vi "Write Close Panel on Exit_.vi"(8 "error in (no error)":errorcluster, 10 "Close Panel on Exit?":bool, 11 "UI ActorTop in":refnum<class "UIActorTop.lvclass">) -> (0 "error out":errorcluster, 3 "UI ActorTop out":refnum<class "UIActorTop.lvclass">)   [LabVIEW 2021, in "AbstractActorTemplate.lvlib" / "UIActorTop.lvclass"]
uses:
  <userlib>/John_Lib/AbstractActorTemplate/AbstractActorTemplate/UIActorTop.lvclass
  <userlib>/John_Lib/AbstractActorTemplate/AbstractActorTemplate/UIActorTop.lvclass/UIActorTop.ctl
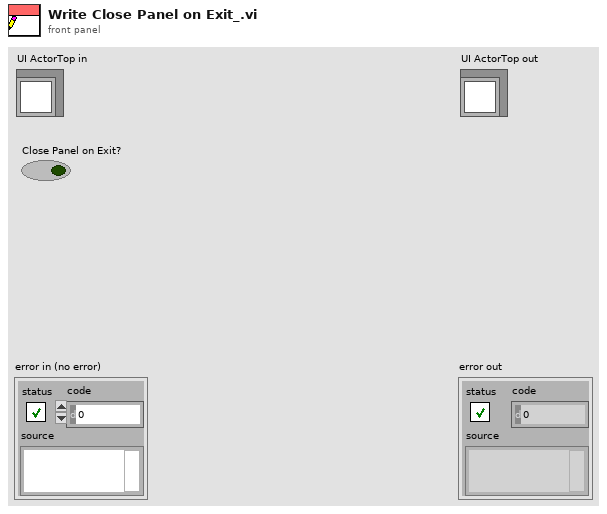
[diagram p1: front panel]
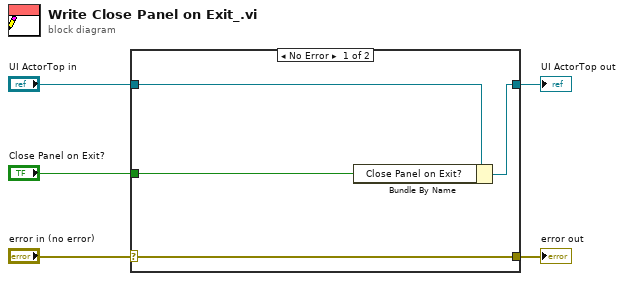
[diagram p0: block diagram]
diagram:
  n1 = case shown="No Error" "error in (no error)" {
    selector: "error in (no error)" -> [w9 w10]
    tunnel: [w9 w10] -> w4
    tunnel: [w7 w11] -> w2
    tunnel: "UI ActorTop in" -> [w8 w11]
    tunnel: "Close Panel on Exit?" -> [w6 _]
    frame No Error {
      n2 = Bundle By Name(cluster=w8, "Close Panel on Exit?"=w6) -> (w7:refnum<class "UIActorTop.lvclass">)
    }
    frame Error {
    }
  }
  "error out" <- w4
  "UI ActorTop out" <- w2
